vi "ABB Noise Analysis.vi"() -> ()   [LabVIEW 2017]
uses:
  ABB global.vi
panel:
  in  "Number Points":i32=12 min=1 max=25 step=1
  in  "Running Average levels (dB)":cluster{"Total":dbl, "Log":dbl}
  in  "Background Average levels (dB)":cluster{"Total":dbl, "Log":dbl}
  in  "Motor Running Noise levels dB(A)":string[][](table)
  in  "Background Noise levels dB(A)":string[][](table)
  out "Serial number":string
  out "W.O number":string
  out "Timedate":string
  in  "Exit":bool
  # "Noise levels"
  # "?"
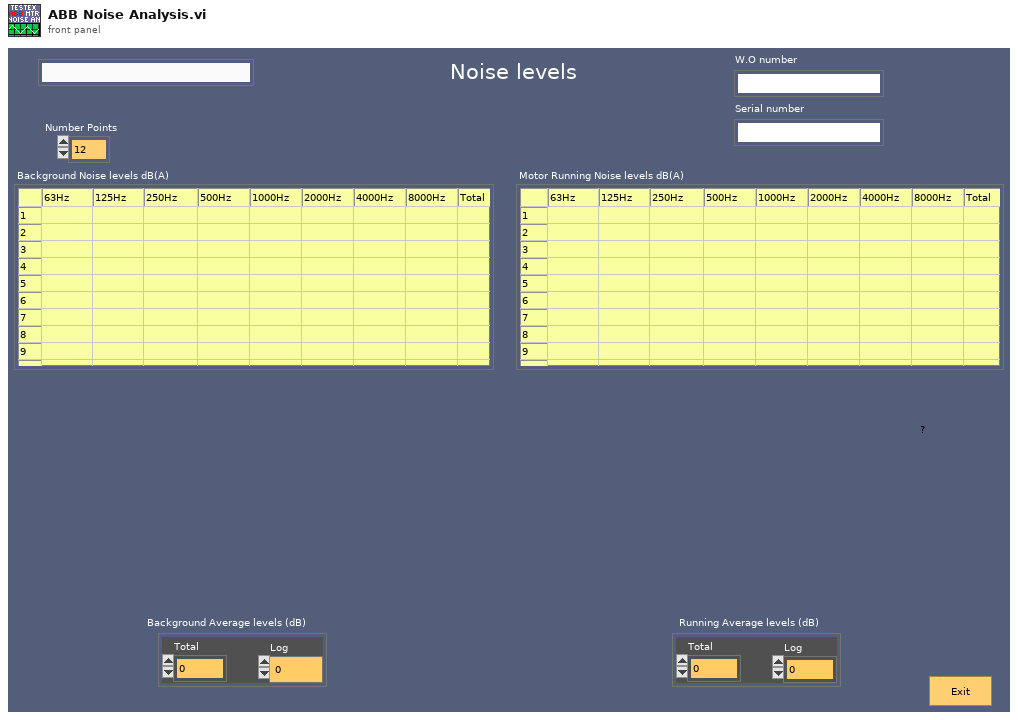
[diagram p1: front panel]
types:
  T1 = cluster{"Simulate Norma":bool, "Norma 5000 Address":u8, "WebDaq IP Address":string, "Simulate cDAQ":bool}
  T2 = cluster{"integer":i32, "Dbl":dbl, "String":string, "Boolean":bool}
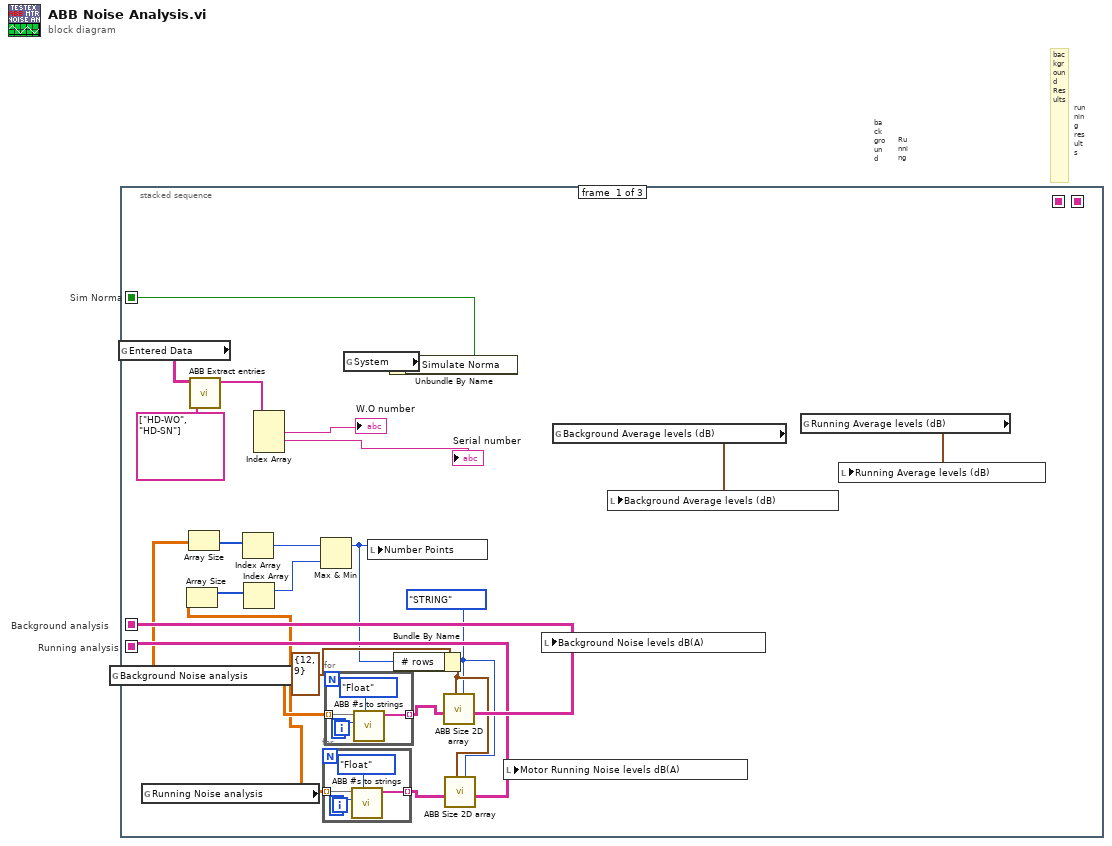
[diagram p0: block diagram]
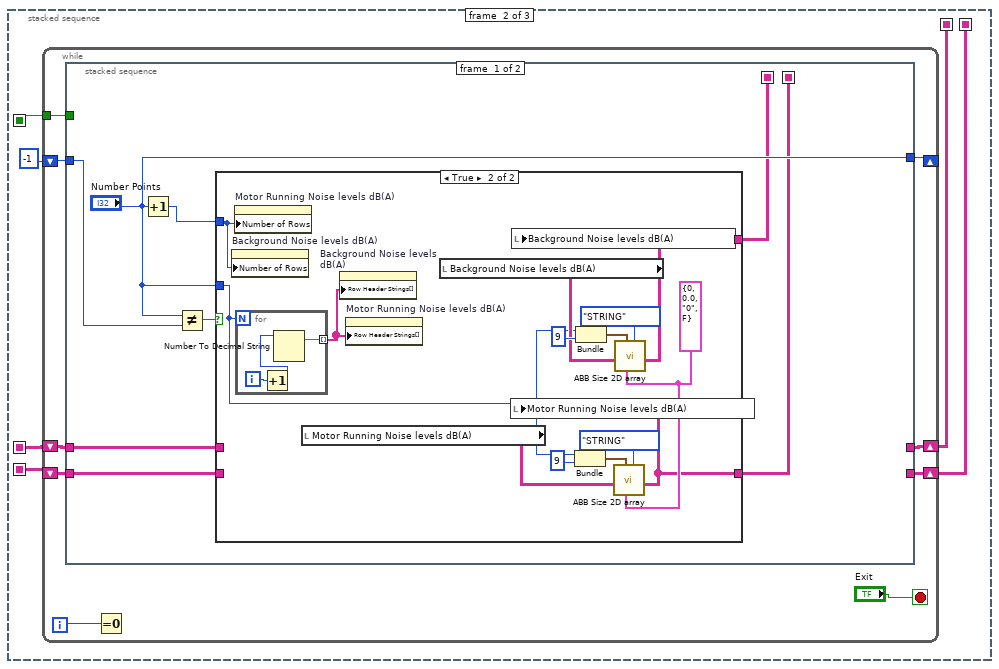
[diagram p2: hidden frame]
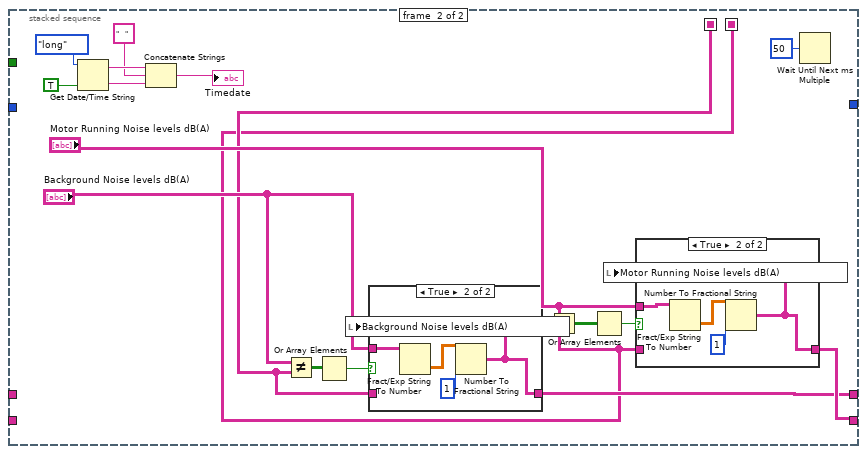
[diagram p4: hidden frame]
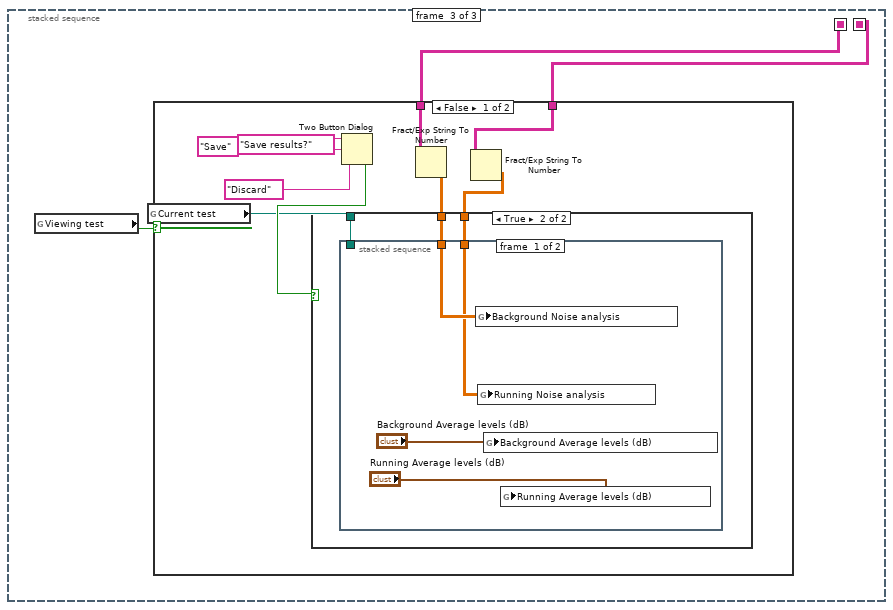
[diagram p7: hidden frame]
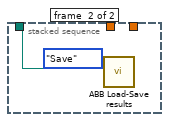
[diagram p9: hidden frame]
diagram:
  # "Running"
  # "background"
  # "running results"
  # "Running analysis"
  # "Sim Norma"
  # "Background analysis"
  # "background Results"
  n1 = stacked-sequence {
    seq-local: [w22 _ _] -> [_ w37 _]
    seq-local: [w9 _ _] -> [_ w36 _]
    seq-local: [_ w35 _] -> [_ _ w102]
    seq-local: [w7 _ _] -> [_ w34 _]
    seq-local: [_ w33 _] -> [_ _ w101]
    frame #0 {
      w1 = enum16{"Integer", "DBL", "STRING", "BOOLEAN"}."STRING" ("Type")
      n2 = global read "ABB global.vi" "Background Noise analysis"() -> (w4:dbl[][])
      n3 = global read "ABB global.vi" "Entered Data"() -> (w21:string[][])
      n4 = global read "ABB global.vi" "Running Noise analysis"() -> (w3:dbl[][])
      n5 = Array Size(array=w3) -> (size(s)=w13:i32[])
      n6 = Array Size(array=w4) -> (size(s)=w14:i32[])
      n7 = call "ABB Extract entries.vi"("Entry IDs"=string[] ["HD-WO", "HD-SN"], "Entry table in"=w21) -> ("Selected Entries"=w20:string[])  [unwired: 9 in]
      n8 = Index Array(array=w14) -> (element=w12:i32)  [unwired: 1 in]
      n9 = Index Array(array=w13) -> (element=w11:i32)  [unwired: 1 in]
      n10 = Index Array(array=w20) -> (element #1=→"W.O number":string, element #2=→"Serial number":string)  [unwired: 3 in, 1 out]
      n11 = Max & Min(x=w12, y=w11) -> (max(x,y)=w2:i32)  [unwired: 1 out]
      n12 = for {
        tunnel: w3 -> [w27] mode=indexing
        tunnel: [w24] -> w8 mode=indexing
        n13 = call "ABB #s to strings.vi"("# type"=enum16{"Float", "Relative time HH:MM"}."Float", "Precision"=3, "Numbers in"=w27) -> ("Strings out"=w24:string[])  [unwired: 8 in]
      }
      n14 = for {
        tunnel: w4 -> [w31] mode=indexing
        tunnel: [w28] -> w10 mode=indexing
        n15 = call "ABB #s to strings.vi"("# type"=enum16{"Float", "Relative time HH:MM"}."Float", "Precision"=3, "Numbers in"=w31) -> ("Strings out"=w28:string[])  [unwired: 8 in]
      }
      n16 = global read "ABB global.vi" "System"() -> (w23:T1)
      n17 = local write "Number Points"(w2) -> ()
      n18 = Unbundle By Name(w23) -> ("Simulate Norma"=w22:bool)
      n19 = Bundle By Name(cluster=cluster{"# rows":i32, "# cols":i32} {"# rows"=12, "# cols"=9} ("Size"), "# rows"=w2) -> (w6:cluster{"# rows":i32, "# cols":i32})
      n20 = call "ABB Size 2D array.vi"("Type"=w1, "Size"=w6, "String Array in"=w10) -> ("String Array out"=w9:string[][])  [unwired: 5 in, 3 out]
      n21 = call "ABB Size 2D array.vi"("Type"=w1, "Size"=w6, "String Array in"=w8) -> ("String Array out"=w7:string[][])  [unwired: 5 in, 3 out]
      n22 = local write "Motor Running Noise levels dB(A)"(w7) -> ()
      n23 = local write "Background Noise levels dB(A)"(w9) -> ()
      n24 = global read "ABB global.vi" "Background Average levels (dB)"() -> (w15:cluster{"Total":dbl, "Log":dbl})
      n25 = local write "Background Average levels (dB)"(w15) -> ()
      n26 = global read "ABB global.vi" "Running Average levels (dB)"() -> (w16:cluster{"Total":dbl, "Log":dbl})
      n27 = local write "Running Average levels (dB)"(w16) -> ()
    }
    frame #1 {
      n28 = while {
        tunnel: w37 -> [w45]
        shift-right: [w43] -> w35
        shift-left: w36 -> [w44]
        shift-right: [w40] -> w33
        shift-left: w34 -> [w41]
        shift-right: [w39] -> _
        shift-left: -1 -> [w38]
        i -> [w42]
        stop <- "Exit" stop-if-true
        n29 = stacked-sequence {
          seq-local: [w48 _] -> [_ w75]
          seq-local: [w47 _] -> [_ w74]
          tunnel: w45 -> [_ _]
          tunnel: [_ w76] -> w43
          tunnel: w44 -> [w50 _]
          tunnel: w41 -> [w49 _]
          tunnel: [_ w79] -> w40
          tunnel: ["Number Points" _] -> w39
          tunnel: w38 -> [w53 _]
          frame #0 {
            n30 = Increment(x="Number Points") -> (x+1=w54:i32)
            n31 = Not Equal?(x="Number Points", y=w53) -> (x != y?=w52:bool)
            n32 = case shown="True" w52 {
              tunnel: "Number Points" -> [_ w60]
              tunnel: w54 -> [_ w67]
              tunnel: w50 -> [w56 _]
              tunnel: w49 -> [w55 _]
              tunnel: [w56 w58] -> w48
              tunnel: [w55 w57] -> w47
              frame False {
              }
              frame True {
                w59 = T2 {"integer"=0, "Dbl"=0.0, "String"="0", "Boolean"=FALSE} ("Defaults")
                n33 = property on="Background Noise levels dB(A)" class="Tbl (strict)"("Number of Rows"=w67) -> ()  [unwired: 2 in, 2 out]
                n34 = property on="Motor Running Noise levels dB(A)" class="Tbl (strict)"("Number of Rows"=w67) -> ()  [unwired: 2 in, 2 out]
                n35 = for {
                  N: w60 -> [_]
                  tunnel: [w71] -> w65 mode=indexing
                  i -> [w73]
                  n36 = Increment(x=w73) -> (x+1=w72:i32)
                  n37 = Number To Decimal String(number=w72) -> (decimal integer string=w71:string)  [unwired: 1 in]
                }
                n38 = local read "Motor Running Noise levels dB(A)"() -> (w64:string[][])
                n39 = property on="Background Noise levels dB(A)" class="Tbl (strict)"("Row Header Strings[]"=w65) -> ()  [unwired: 2 in, 2 out]
                n40 = property on="Motor Running Noise levels dB(A)" class="Tbl (strict)"("Row Header Strings[]"=w65) -> ()  [unwired: 2 in, 2 out]
                n41 = local read "Background Noise levels dB(A)"() -> (w66:string[][])
                n42 = Bundle("Number Points"=w60, 9) -> (w62:cluster{"Number Points":i32, i32})  [unwired: 1 in]
                n43 = Bundle("Number Points"=w60, 9) -> (w69:cluster{"Number Points":i32, i32})  [unwired: 1 in]
                n44 = call "ABB Size 2D array.vi"("Type"=enum16{"Integer", "DBL", "STRING", "BOOLEAN"}."STRING", "Defaults"=w59, "Size"=w62, "String Array in"=w64) -> ("String Array out"=w57:string[][])  [unwired: 4 in, 3 out]
                n45 = local write "Motor Running Noise levels dB(A)"(w57) -> ()
                n46 = call "ABB Size 2D array.vi"("Type"=enum16{"Integer", "DBL", "STRING", "BOOLEAN"}."STRING", "Defaults"=w59, "Size"=w69, "String Array in"=w66) -> ("String Array out"=w58:string[][])  [unwired: 4 in, 3 out]
                n47 = local write "Background Noise levels dB(A)"(w58) -> ()
              }
            }
          }
          frame #1 {
            n48 = Get Date/Time String(date format (0)=enum16{"short", "long", "abbreviated"}."long", want seconds? (F)=TRUE) -> (date string=w88:string, time string=w87:string)  [unwired: 1 in]
            n49 = Concatenate Strings(w88, "   ", w87) -> (→"Timedate":string)
            n50 = Not Equal?(x="Background Noise levels dB(A)", y=w75) -> (x != y?=w83:bool[][])
            n51 = Or Array Elements(Boolean array=w83) -> (logical OR=w82:bool)
            n52 = case shown="True" w82 {
              tunnel: w75 -> [w96 _]
              tunnel: [w96 w98] -> w76
              tunnel: "Background Noise levels dB(A)" -> [_ w97]
              frame False {
              }
              frame True {
                n53 = Fract/Exp String To Number(string=w97) -> (number=w100:dbl[][])  [unwired: 3 in, 1 out]
                n54 = Number To Fractional String(number=w100, precision (6)=i16 1) -> (F-format string=w98:string[][])  [unwired: 2 in]
                n55 = local write "Background Noise levels dB(A)"(w98) -> ()
              }
            }
            n56 = Not Equal?(x="Motor Running Noise levels dB(A)", y=w74) -> (x != y?=w81:bool[][])
            n57 = Or Array Elements(Boolean array=w81) -> (logical OR=w80:bool)
            n58 = case shown="True" w80 {
              tunnel: w74 -> [w91 _]
              tunnel: [w91 w93] -> w79
              tunnel: "Motor Running Noise levels dB(A)" -> [_ w92]
              frame False {
              }
              frame True {
                n59 = Fract/Exp String To Number(string=w92) -> (number=w95:dbl[][])  [unwired: 3 in, 1 out]
                n60 = Number To Fractional String(number=w95, precision (6)=i16 1) -> (F-format string=w93:string[][])  [unwired: 2 in]
                n61 = local write "Motor Running Noise levels dB(A)"(w93) -> ()
              }
            }
            n62 = Wait Until Next ms Multiple(millisecond multiple=u32 50) -> ()  [unwired: 1 out]
          }
        }
        n63 = Equal To 0?(x=w42) -> ()  [unwired: 1 out]
      }
    }
    frame #2 {
      n64 = global read "ABB global.vi" "Viewing test"() -> (w103:bool)
      n65 = case shown="False" w103 {
        tunnel: w102 -> [w109 _]
        tunnel: w101 -> [w105 _]
        frame False {
          n66 = global read "ABB global.vi" "Current test"() -> (w110:path)
          n67 = Two Button Dialog(message="Save results?", 1:"Discard" ("F button name (\"Cancel\")"), 2:"Save" ("T button name (\"OK\")")) -> (T button?=w111:bool)
          n68 = Fract/Exp String To Number(string=w109) -> (number=w108:dbl[][])  [unwired: 3 in, 1 out]
          n69 = Fract/Exp String To Number(string=w105) -> (number=w104:dbl[][])  [unwired: 3 in, 1 out]
          n70 = case shown="True" w111 {
            tunnel: w108 -> [_ w115]
            tunnel: w110 -> [_ w114]
            tunnel: w104 -> [_ w113]
            frame False {
            }
            frame True {
              n71 = stacked-sequence {
                tunnel: w115 -> [w119 _]
                tunnel: w114 -> [_ w120]
                tunnel: w113 -> [w118 _]
                frame #0 {
                  n72 = global write "ABB global.vi" "Background Noise analysis"(w119) -> ()
                  n73 = global write "ABB global.vi" "Running Noise analysis"(w118) -> ()
                  n74 = global write "ABB global.vi" "Background Average levels (dB)"("Background Average levels (dB)") -> ()
                  n75 = global write "ABB global.vi" "Running Average levels (dB)"("Running Average levels (dB)") -> ()
                }
                frame #1 {
                  n76 = call "ABB Load-Save results.vi"("Path"=w120, "Mode"=enum16{"LOAD", "Save"}."Save") -> ()  [unwired: 10 in]
                }
              }
            }
          }
        }
        frame True {
        }
      }
    }
  }
